vi "SI8.vi"(4 "error in":T13, 7 "Command":T14) -> (0 "error out":T13, 3 "Response":T11)   [LabVIEW 2018]
uses:
  MOKO_LabViewLibrary/MokoLowLevel/MokoLowLovelControl/MLLC_Command.ctl
  MOKO_LabViewLibrary/MokoLowLevel/MokoLowLovelControl/MLLC_Error.ctl
  MOKO_LabViewLibrary/MokoLowLevel/MokoLowLovelControl/MLLC_Mode.ctl
  MOKO_LabViewLibrary/MokoLowLevel/MokoLowLovelControl/MLLC_Response.ctl
  MOKO_LabViewLibrary/MokoLowLevel/MokoLowLovelControl/MLLC_DriverName.ctl
  MOKO_LabViewLibrary/MokoLowLevel/MokoLowLovelControl/MLLC_ResponseInit.ctl
  MOKO_LabViewLibrary/MokoLowLevel/MokoLowLovelControl/MLLC_Request.ctl
  MOKO_LabViewLibrary/MokoLowLevel/MokoLowLovelControl/MLLC_ErrorCode.ctl
  MOKO_LabViewLibrary/MokoLowLevel/MokoLowLovelControl/MLLC_ConnectCluster.ctl
  MOKO_LabViewLibrary/MokoLowLevel/MokoLowLovelControl/MLLC_InterfaceType.ctl
  MOKO_LabViewLibrary/MokoLowLevel/MokoLowLovelControl/MLLC_OpenedSession.ctl
  MOKO_LabViewLibrary/MokoLowLevel/MokoLowLovelControl/MLLC_InterfaceSettings.ctl
  MOKO_LabViewLibrary/MokoLowLevel/MokoLowLovelControl/MLLC_InterfaceKind.ctl
  MOKO_LabViewLibrary/MokoLowLevel/MokoLowLovelControl/MLLC_Rs232Settings.ctl
panel:
  in  "Settings":T6={"Permanent data"={"Connect"={"InterfaceType"=enum."VISA", "OpenedSession"="COM4", "InterfaceSettings"={"Interface"=enum."RS232", "EOS 4 read"=enum."Default (=EOS 4 write)", "EOS 4 write"=enum."CR (\\r)", "TMO, ms"=2000, "Sett"=variant(cluster{"Baud Rate":u32, "Data Bits":u16, "Parity":u16, "Stop Bits":u16, "Flow Control":u16, "Eho":bool} {"Baud Rate"=75, "Data Bits"=0, "Parity"=0, "Stop Bits"=0, "Flow Control"=0, "Eho"=FALSE})}}}, "Saved Data"=variant}
  in  "Error Code":T7=5420
  in  "Request":T8="?MOD"
  in  "ResponseInit":T9="XP2I"
  in  "Driver Name":T10="Crystal XP2"
  in  "Mode":T12=enum."Check"
  # "SI8"
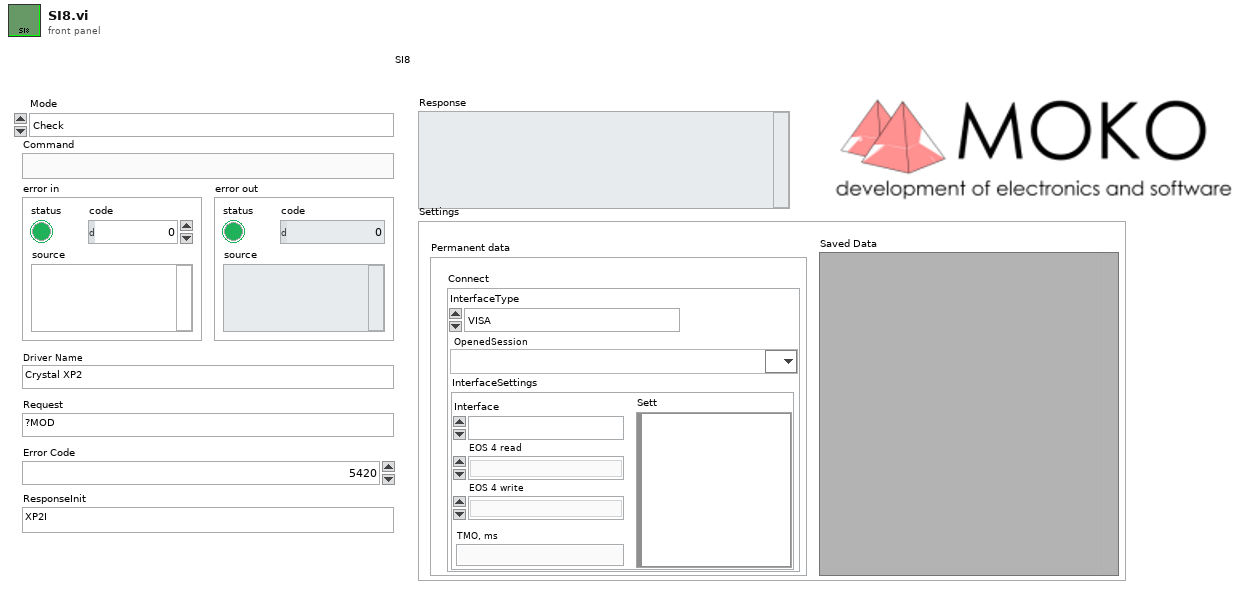
[diagram p1: front panel]
types:
  T1 = typedef "MLLC_ConnectCluster.ctl" = cluster{"InterfaceType":T2, "OpenedSession":T3, "InterfaceSettings":T4}
  T2 = typedef "MLLC_InterfaceType.ctl" = enum16{"VISA", "Prologix USB-GPIB"}
  T3 = typedef "MLLC_OpenedSession.ctl" = refnum<visa-resource-name>
  T4 = typedef "MLLC_InterfaceSettings.ctl" = cluster{"Interface":T5, "EOS 4 read":enum16{"Default (=EOS 4 write)", "CR (\\r)", "LF (\\n)", "None"}, "EOS 4 write":enum16{"CR+LF (\\r\\n)", "CR (\\r)", "LF (\\n)", "None"}, "TMO, ms":i32, "Sett":variant}
  T5 = typedef "MLLC_InterfaceKind.ctl" = enum16{"RS232", "GPIB", "USB", "Ethernet", "another"}
  T6 = cluster{"Permanent data":cluster{"Connect":T1}, "Saved Data":variant}
  T7 = typedef "MLLC_ErrorCode.ctl" = u32
  T8 = typedef "MLLC_Request.ctl" = string
  T9 = typedef "MLLC_ResponseInit.ctl" = string
  T10 = typedef "MLLC_DriverName.ctl" = string
  T11 = typedef "MLLC_Response.ctl" = string
  T12 = typedef "MLLC_Mode.ctl" = enum16{"get", "set", "close", "Init", "Check"}
  T13 = typedef "MLLC_Error.ctl" = errorcluster
  T14 = typedef "MLLC_Command.ctl" = string
  T15 = typedef "MLLC_Rs232Settings.ctl" = cluster{"Baud Rate":u32, "Data Bits":u16, "Parity":u16, "Stop Bits":u16, "Flow Control":u16, "Eho":bool}
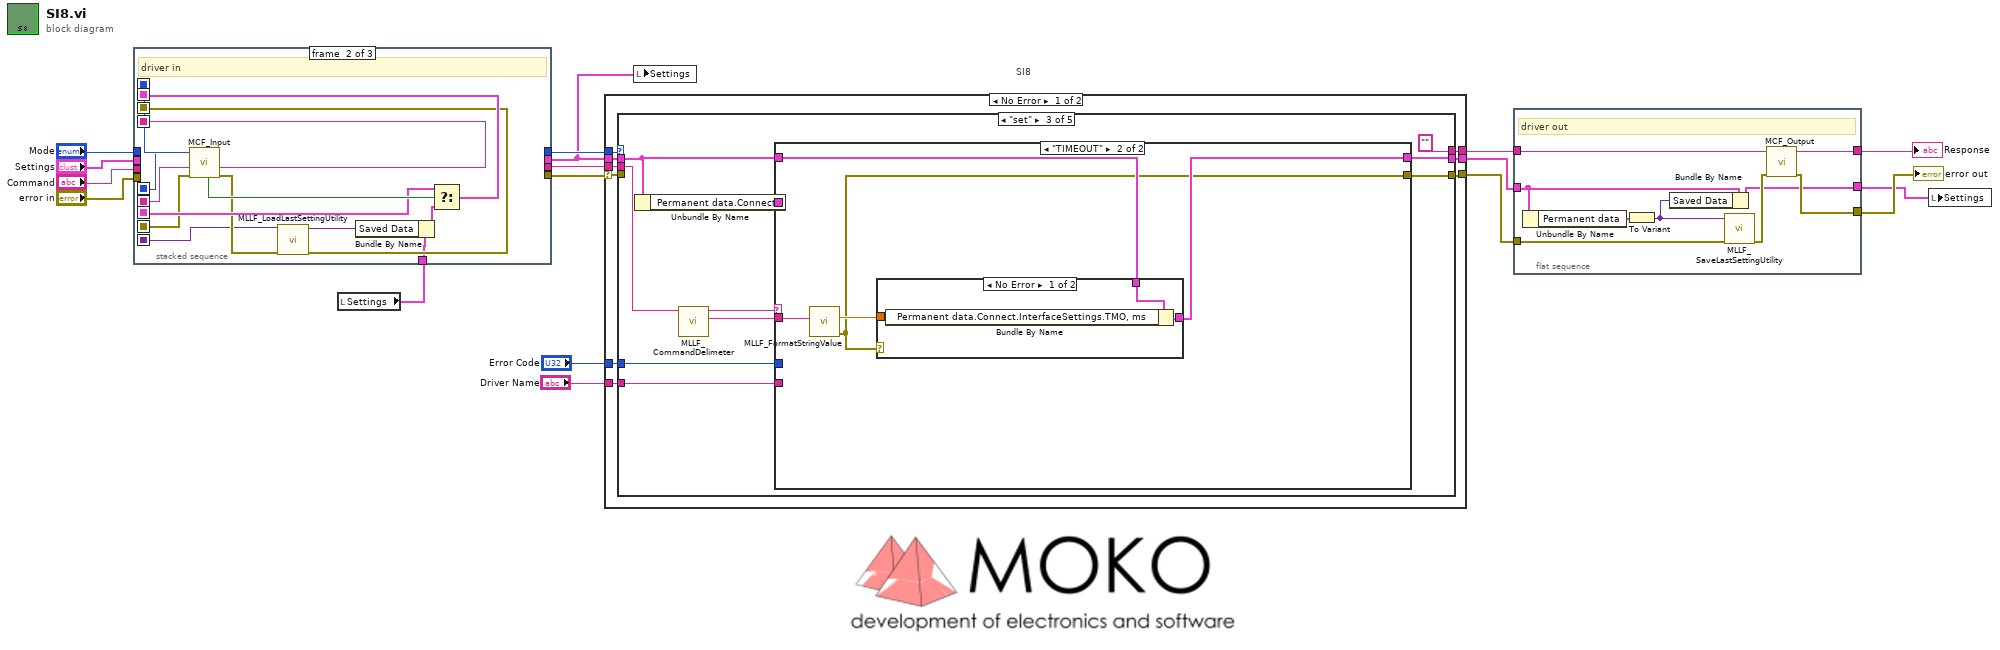
[diagram p0: block diagram]
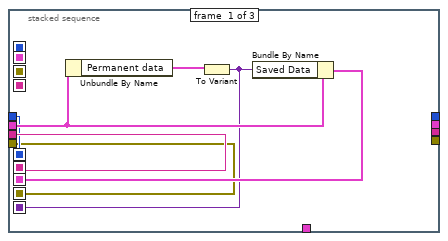
[diagram p2: hidden frame]
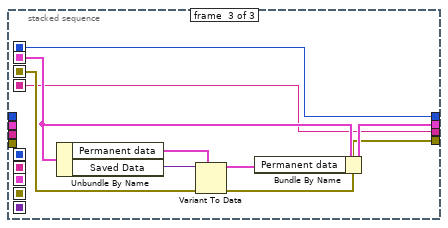
[diagram p3: hidden frame]
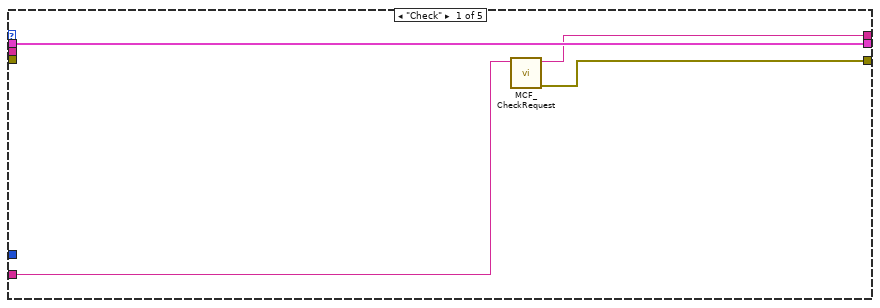
[diagram p4: hidden frame]
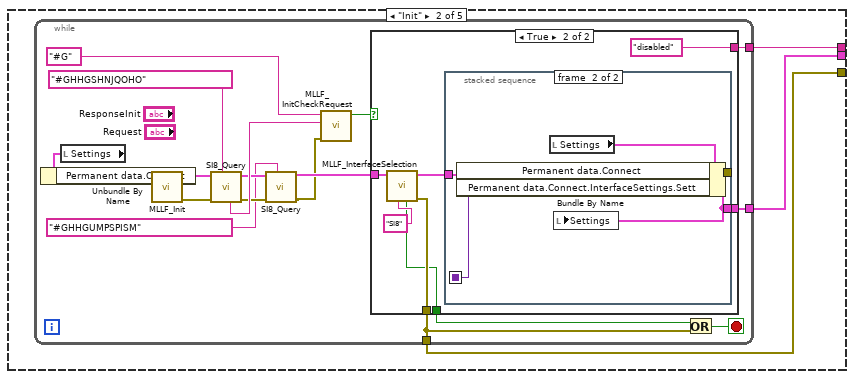
[diagram p5: hidden frame]
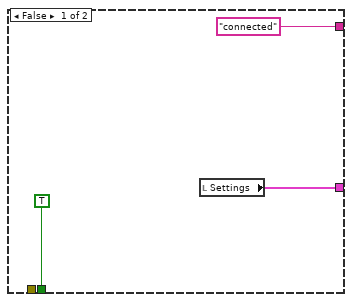
[diagram p6: hidden frame]
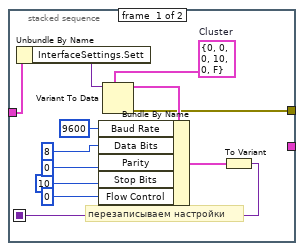
[diagram p7: hidden frame]
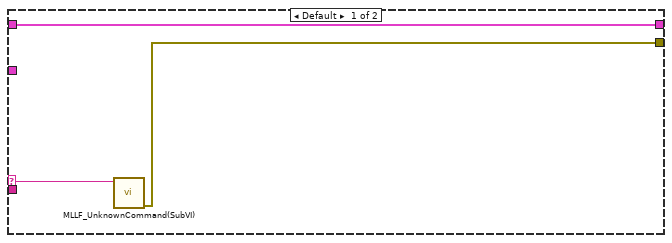
[diagram p8: hidden frame]
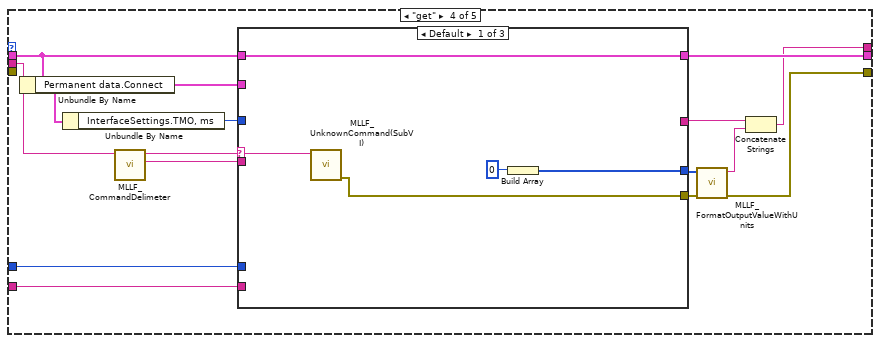
[diagram p10: hidden frame]
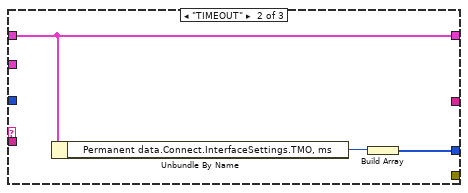
[diagram p11: hidden frame]
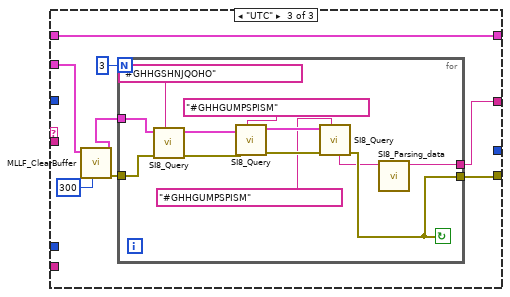
[diagram p12: hidden frame]
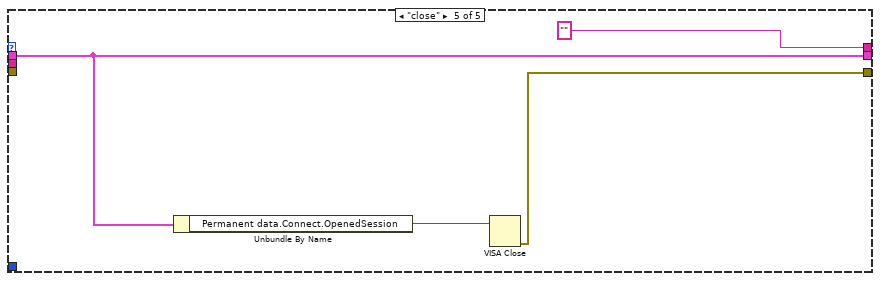
[diagram p13: hidden frame]
diagram:
  # "SI8"
  n1 = local read "Settings"() -> (w7:T6)
  n2 = stacked-sequence {
    seq-local: [w20 _ _] -> [_ w36 _]
    seq-local: [w19 _ _] -> [_ w37 _]
    seq-local: [w22 _ _] -> [_ w32 _]
    seq-local: [w18 _ _] -> [_ w31 _]
    seq-local: [w21 _ _] -> [_ w27 _]
    seq-local: [_ w28 _] -> [_ _ w44]
    seq-local: [_ w38 _] -> [_ _ w41]
    seq-local: [_ w35 _] -> [_ _ w40]
    seq-local: [_ w34 _] -> [_ _ w45]
    tunnel: "Command" -> [w20 _ _]
    tunnel: "Mode" -> [w19 _ _]
    tunnel: "error in" -> [w18 _ _]
    tunnel: "Settings" -> [w23 _ _]
    tunnel: w7 -> [_ w26 _]
    tunnel: [_ _ w40] -> w9
    tunnel: [_ _ w43] -> w10
    tunnel: [_ _ w42] -> w8
    tunnel: [_ _ w41] -> w11
    frame #0 {
      n3 = Unbundle By Name(w23) -> ("Permanent data"=w24:cluster{"Connect":T1})
      n4 = To Variant(anything=w24) -> (Variant=w21:variant)
      n5 = Bundle By Name(cluster=w23, "Saved Data"=w21) -> (w22:T6)
    }
    frame #1 {
      # "driver in"
      n6 = call "MCF_Input.vi"("Error In"=w31, "Command in"=w36, "Mode in"=w37) -> ("Error Out"=w30:errorcluster, "Command out"=w35:string, "Mode out"=w38:T12, "Boolean"=w33:bool)  [unwired: 5 in]
      n7 = call "MLLF_LoadLastSettingUtility.vi"("Error In"=w30, "Save data in"=w27) -> ("Error Out"=w28:errorcluster, "Save data out"=w25:variant)  [unwired: 8 in]
      n8 = Bundle By Name(cluster=w26, "Saved Data"=w25) -> (w29:T6)
      n9 = Select(t=w32, s=w33, f=w29) -> (s? t:f=w34:T6)
    }
    frame #2 {
      n10 = Unbundle By Name(w45) -> ("Permanent data"=w46:cluster{"Connect":T1}, "Saved Data"=w39:variant)
      n11 = Variant To Data(error in=w44, type=w46, Variant=w39) -> (data=w47:cluster{"Connect":T1}, error out=w42:errorcluster)
      n12 = Bundle By Name(cluster=w45, "Permanent data"=w47) -> (w43:T6)
    }
  }
  n13 = case shown="No Error" w8 {
    selector: w8 -> [w53 w178]
    tunnel: [w48 w178] -> w4
    tunnel: w11 -> [w56 _]
    tunnel: [w55 _] -> w6
    tunnel: w9 -> [w54 _]
    tunnel: w10 -> [w50 w177]
    tunnel: "Error Code" -> [w52 _]
    tunnel: "Driver Name" -> [w51 _]
    tunnel: [w49 w177] -> w5
    frame No Error {
      n14 = case shown="\"set\"" w56 {
        tunnel: [w58 w63 "" ("Output String") w131 "" ("Output String")] -> w55
        tunnel: w54 -> [_ _ w111 w135 _]
        tunnel: w53 -> [_ _ _ _ _]
        tunnel: w52 -> [_ _ w117 w143 _]
        tunnel: w51 -> [w59 _ w114 w142 _]
        tunnel: w50 -> [w60 _ w116 w144 w175]
        tunnel: [w60 w62 w115 w141 w175] -> w49
        tunnel: [w57 w61 w108 w130 w174] -> w48
        frame "Check" {
          n15 = call "MCF_CheckRequest.vi"("Driver Name"=w59) -> ("Error Out"=w57:errorcluster, "Output String"=w58:string)  [unwired: 9 in]
        }
        frame "Init" {
          n16 = while {
            tunnel: [w78] -> w61
            tunnel: [w77] -> w63
            tunnel: [w76] -> w62
            stop <- w80 stop-if-true
            n17 = local read "Settings"() -> (w74:T6)
            n18 = Unbundle By Name(w74) -> ("Permanent data.Connect"=w73:T1)
            n19 = call "MLLF_Init.vi"("DriverConnect in"=w73) -> ("Error Out"=w81:errorcluster, "DriverConnect out"=w71:T1)  [unwired: 7 in]
            n20 = call "SI8_Query.vi"("String"="#GHHGSHNJQOHO", "error in (no error)"=w81, "DriverConnect in"=w71) -> ("error out"=w68:errorcluster, "DriverConnect out"=w67:T1, "String from device out"=w69:string)  [unwired: 6 in]
            n21 = call "SI8_Query.vi"("String"="#GHHGUMPSPISM", "error in (no error)"=w68, "DriverConnect in"=w67) -> ("error out"=w64:errorcluster, "DriverConnect out"=w65:T1)  [unwired: 6 in, 1 out]
            n22 = call "MLLF_InitCheckRequest.vi"("error in (no error)"=w64, "Answer"=w69, "Response Init"="#G") -> ("Design"=w75:bool)  [unwired: 5 in, 3 out]
            n23 = case shown="True" w75 {
              tunnel: w65 -> [_ w90]
              tunnel: [TRUE w86] -> w79
              tunnel: [_ w91] -> w78
              tunnel: ["connected" "disabled"] -> w77
              tunnel: [w82 w85] -> w76
              frame False {
                n24 = local read "Settings"() -> (w82:T6)
              }
              frame True {
                n25 = call "MLLF_InterfaceSelection.vi"("Driver Name"="SI8" ("String"), "DriverConnect in"=w90) -> ("error out"=w91:T13, "DriverConnect out"=w89:T1, "stop init?"=w86:bool)  [unwired: 7 in]
                n26 = stacked-sequence {
                  seq-local: [w95 _] -> [_ w104]
                  tunnel: w89 -> [w93 w105]
                  tunnel: [w96 _] -> _
                  tunnel: [_ w106] -> w85
                  frame #0 {
                    w97 = T15 {"Baud Rate"=0, "Data Bits"=0, "Parity"=0, "Stop Bits"=10, "Flow Control"=0, "Eho"=FALSE}  # Cluster
                    # "перезаписываем настройки"
                    n27 = Unbundle By Name(w93) -> ("InterfaceSettings.Sett"=w92:variant)
                    n28 = Variant To Data(type=w97, Variant=w92) -> (data=w98:T15, error out=w96:errorcluster)  [unwired: 1 in]
                    n29 = Bundle By Name(cluster=w98, "Baud Rate"=u32 9600, "Data Bits"=u16 8 ("Serial Settings:Data Bits"), "Parity"=u16 0 ("Serial Settings:Parity"), "Stop Bits"=u16 10 ("Serial Settings:Stop Bits"), "Flow Control"=u16 0 ("Serial Settings:Flow Control")) -> (w103:T15)
                    n30 = To Variant(anything=w103) -> (Variant=w95:variant)
                  }
                  frame #1 {
                    n31 = local read "Settings"() -> (w107:T6)
                    n32 = Bundle By Name(cluster=w107, "Permanent data.Connect"=w105, "Permanent data.Connect.InterfaceSettings.Sett"=w104) -> (w106:T6)
                    n33 = local write "Settings"(w106) -> ()
                  }
                }
              }
            }
            n34 = Or(x=w79, y=w78) -> (x .or. y?=w80:bool)
          }
        }
        frame "set" {
          n35 = Unbundle By Name(w116) -> ("Permanent data.Connect"=w112:T1)
          n36 = call "MLLF_CommandDelimeter.vi"("command with param"=w111) -> ("param 1"=w109:string, "command"=w110:string)  [unwired: 6 in, 3 out]
          n37 = case shown="\"TIMEOUT\"" w110 {
            selector: w110 -> [w119 _]
            tunnel: w109 -> [_ w123]
            tunnel: w117 -> [_ _]
            tunnel: w116 -> [w120 w124]
            tunnel: [w120 w125] -> w115
            tunnel: w114 -> [_ _]
            tunnel: [w118 w121] -> w108
            tunnel: w112 -> [_ _]
            frame Default {
              n38 = call "MLLF_UnknownCommand(SubVI).vi"("Unknown command"=w119) -> ("error out"=w118:errorcluster)  [unwired: 10 in]
            }
            frame "TIMEOUT" {
              n39 = call "MLLF_FormatStringValue.vi"("String Value"=w123) -> ("error out"=w121:T13, "number"=w122:dbl)  [unwired: 8 in, 1 out]
              n40 = case shown="No Error" w121 {
                tunnel: [w128 w129] -> w125
                tunnel: w124 -> [w127 w129]
                tunnel: w122 -> [w126 _]
                frame No Error {
                  n41 = Bundle By Name(cluster=w127, "Permanent data.Connect.InterfaceSettings.TMO, ms"=w126) -> (w128:T6)
                }
                frame Error {
                }
              }
            }
          }
        }
        frame "get" {
          n42 = Unbundle By Name(w144) -> ("Permanent data.Connect"=w134:T1)
          n43 = Unbundle By Name(w134) -> ("InterfaceSettings.TMO, ms"=w138:i32)
          n44 = call "MLLF_CommandDelimeter.vi"("command with param"=w135) -> ("param 1"=w132:string, "command"=w133:string)  [unwired: 6 in, 3 out]
          n45 = case shown="Default" w133 {
            selector: w133 -> [w146 _ _]
            tunnel: w132 -> [_ _ _]
            tunnel: [w145 _ w157] -> w140
            tunnel: w143 -> [_ _ _]
            tunnel: [w149 w152 w160] -> w141
            tunnel: w144 -> [w149 w152 w160]
            tunnel: [w147 w150 _] -> w139
            tunnel: w142 -> [_ _ _]
            tunnel: w138 -> [_ _ _]
            tunnel: [_ _ w159] -> w136
            tunnel: w134 -> [_ _ w156]
            frame Default {
              n46 = call "MLLF_UnknownCommand(SubVI).vi"("Unknown command"=w146) -> ("error out"=w145:errorcluster)  [unwired: 10 in]
              n47 = Build Array(0 ("TimeOut")) -> (w147:i32[])
            }
            frame "TIMEOUT" {
              n48 = Unbundle By Name(w152) -> ("Permanent data.Connect.InterfaceSettings.TMO, ms"=w151:i32)
              n49 = Build Array(w151) -> (w150:i32[])
            }
            frame "UTC" {
              n50 = call "MLLF_ClearBuffer.vi"("Timeout"=u32 300, "DriverConnect in"=w156) -> ("Error Out"=w153:errorcluster, "DriverConnect out"=w154:T1)  [unwired: 6 in, 1 out]
              n51 = for {
                N: 3 -> [_]
                tunnel: w154 -> [w172]
                tunnel: [w162] -> w159
                tunnel: [w164] -> w157
                tunnel: w153 -> [w161]
                stop <- w164 continue-if-true
                n52 = call "SI8_Query.vi"("String"="#GHHGSHNJQOHO", "error in (no error)"=w161, "DriverConnect in"=w172) -> ("error out"=w170:errorcluster, "DriverConnect out"=w169:T1)  [unwired: 6 in, 1 out]
                n53 = call "SI8_Query.vi"("String"="#GHHGUMPSPISM", "error in (no error)"=w170, "DriverConnect in"=w169) -> ("error out"=w168:errorcluster, "DriverConnect out"=w167:T1)  [unwired: 6 in, 1 out]
                n54 = call "SI8_Query.vi"("String"="#GHHGUMPSPISM", "error in (no error)"=w168, "DriverConnect in"=w167) -> ("error out"=w164:errorcluster, "String from device out"=w163:string)  [unwired: 6 in, 1 out]
                n55 = call "SI8_Parsing_data.vi"("IN"=w163) -> ("OUT"=w162:string)  [unwired: 10 in]
              }
            }
          }
          n56 = call "MLLF_FormatOutputValueWithUnits.vi"("error in"=w140, "ValuesIn"=w139) -> ("error out"=w130:T13, "Result string"=w137:T14)  [unwired: 8 in]
          n57 = Concatenate Strings(w136, w137) -> (w131:string)
        }
        frame "close" {
          n58 = Unbundle By Name(w175) -> ("Permanent data.Connect.OpenedSession"=w176:T3)
          n59 = VISA Close(VISA resource name=w176) -> (error out=w174:errorcluster)  [unwired: 1 in]
        }
      }
    }
    frame Error {
    }
  }
  n60 = local write "Settings"(w10) -> ()
  n61 = flat-sequence {
    tunnel: [w187] -> w3
    tunnel: [w186] -> w2
    tunnel: w6 -> [w185]
    tunnel: w4 -> [w184]
    tunnel: w5 -> [w180]
    tunnel: [w182] -> w1
    frame #0 {
      # "driver out"
      n62 = Unbundle By Name(w180) -> ("Permanent data"=w179:cluster{"Connect":T1})
      n63 = To Variant(anything=w179) -> (Variant=w181:variant)
      n64 = Bundle By Name(cluster=w180, "Saved Data"=w181) -> (w182:T6)
      n65 = call "MLLF_SaveLastSettingUtility.vi"("error in"=w184, "Saved Data"=w181) -> ("error out"=w183:T13)  [unwired: 8 in, 1 out]
      n66 = call "MCF_Output.vi"("Error In"=w183, "Input"=w185) -> ("Error Out"=w186:errorcluster, "Output"=w187:string)  [unwired: 8 in]
    }
  }
  n67 = local write "Settings"(w1) -> ()
  "error out" <- w2
  "Response" <- w3
